vi "Asynchronously Execute Python Optimization (On-Grid).vi"(8 "error in":errorcluster, 10 "Stop Notifier":refnum<notifier>, 11 "On-Grid in":refnum<class "On-Grid.lvclass">) -> (0 "error out":errorcluster, 3 "On-Grid out":refnum<class "On-Grid.lvclass">)   [LabVIEW 2018, in "On-Grid Actor.lvlib" / "On-Grid.lvclass"]
uses:
  On-Grid.lvclass
  C:/Users/Administrator/Desktop/LabVIEW EMS/Optimization/Generic Optimization Actor/Generic Optimization/Generic Optimization.lvclass
  Global Variables/Global Variables.vi
  Generic Optimization Actor/Generic Optimization/Generic Optimization.lvclass
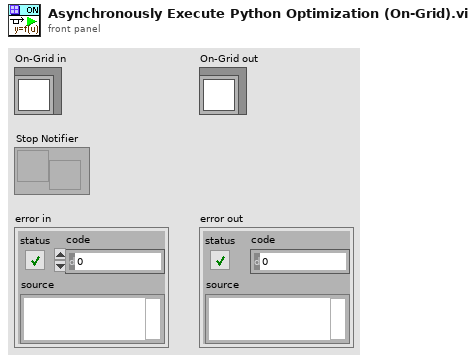
[diagram p1: front panel]
types:
  T1 = typedef "Optimization Type Selector.ctl" = enum16{"Invalid", "Single Phase", "Volttron"}
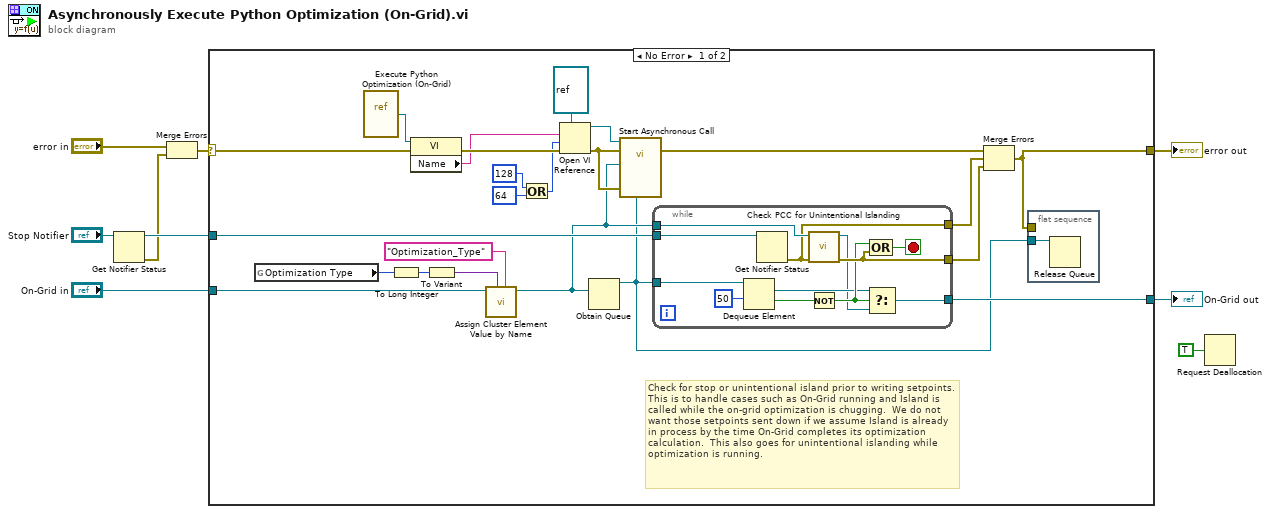
[diagram p0: block diagram]
diagram:
  n1 = Get Notifier Status(notifier="Stop Notifier") -> (notifier out=w5:refnum<notifier>, error out=w3:errorcluster)  [unwired: 1 in, 3 out]
  n2 = Merge Errors("error in", w3) -> (w2:errorcluster)
  n3 = case shown="No Error" w2 {
    selector: w2 -> [w32 w47]
    tunnel: w5 -> [w31 _]
    tunnel: [w30 w47] -> w9
    tunnel: "On-Grid in" -> [w16 w46]
    tunnel: [w14 w46] -> w7
    frame No Error {
      # "Check for stop or unintentional island prior to writing setpoints.  This is to handle cases such as On-Grid running and Island is called while the on-grid optimization is chugging.  We do not want those setpoints sent down if we assume Island is already in process by the time On-Grid completes its optimization calculation.  This also goes for unintentional islanding while optimization is running."
      n4 = global read "Global Variables.vi" "Optimization Type"() -> (w28:T1)
      n5 = vi-ref "Execute Python Optimization (On-Grid).vi"() -> (w20:refnum<vi>)
      n6 = To Long Integer(number=w28) -> (32bit integer=w29:i32)
      n7 = property class="VI"(reference=w20, error in=w32) -> (error out=w22:errorcluster, "Name"=w21:string)  [unwired: 1 out]
      n8 = To Variant(anything=w29) -> (Variant=w27:variant)
      n9 = call "Assign Cluster Element Value by Name.vi"("Element Name"="Optimization_Type" ("Keyword Name"), "Value"=w27, "Generic Optimization"=w16) -> ("Generic Optimization out"=w15:refnum<class "On-Grid.lvclass">)  [unwired: 7 in, 1 out]
      n10 = Or(x=128 ("options"), y=64 ("options")) -> (x .or. y?=w11:i32)
      n11 = Open VI Reference(type specifier VI Refnum (for type only)=refnum<vi> refnum, vi path=w21, options=w11, error in (no error)=w22) -> (vi reference=w25:refnum<vi>, error out=w23:errorcluster)  [unwired: 2 in]
      n12 = Obtain Queue(element data type=w15) -> (queue out=w10:refnum<queue>)  [unwired: 4 in, 2 out]
      n13 = call-by-ref "Start Asynchronous Call"(reference=w25, error in=w23, "Results Queue"=w10, "error in"=w23, "On-Grid in"=w15) -> (error out=w24:errorcluster)  [unwired: 7 in, 3 out]
      n14 = while {
        tunnel: w31 -> [w45]
        tunnel: [w40] -> w17
        tunnel: w10 -> [w44]
        tunnel: w15 -> [w41]
        tunnel: [w34] -> w14
        tunnel: [w39] -> w18
        stop <- w38 stop-if-true
        n15 = Dequeue Element(queue=w44, timeout in ms (-1)=50) -> (element=w36:refnum<class "On-Grid.lvclass">, timed out?=w42:bool)  [unwired: 1 in, 2 out]
        n16 = Get Notifier Status(notifier=w45) -> (error out=w39:errorcluster)  [unwired: 1 in, 4 out]
        n17 = call "Check PCC for Unintentional Islanding.vi"("error in"=w39, "On-Grid in"=w41) -> ("error out"=w40:errorcluster, "On-Grid out"=w35:refnum<class "On-Grid.lvclass">)  [unwired: 8 in]
        n18 = Not(x=w42) -> (.not. x?=w37:bool)
        n19 = Select(t=w36, s=w37, f=w35) -> (s? t:f=w34:refnum<class "On-Grid.lvclass">)
        n20 = Compound Arithmetic op=OR(w37, w40) -> (w38:bool)
      }
      n21 = Merge Errors(w24, w18, w17) -> (w30:errorcluster)
      n22 = flat-sequence {
        tunnel: w10 -> [w33]
        tunnel: w30 -> [_]
        frame #0 {
          n23 = Release Queue(queue=w33) -> ()  [unwired: 2 in, 3 out]
        }
      }
    }
    frame Error {
    }
  }
  "error out" <- w9
  "On-Grid out" <- w7
  n24 = Request Deallocation(TRUE ("flag")) -> ()
